vi "test.vi"() -> ()   [LabVIEW 2012]
panel:
  out "x/y":sgl
  in  "数值 2":sgl
  in  "数值":sgl
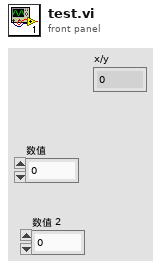
[diagram p1: front panel]
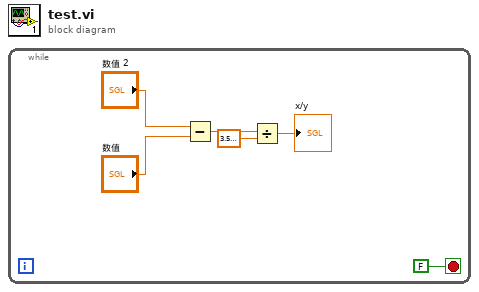
[diagram p0: block diagram]
diagram:
  n1 = while {
    stop <- FALSE stop-if-true
    n2 = Subtract(x="数值 2", y="数值") -> (x-y=w3:sgl)
    n3 = Divide(x=w3, y=sgl 3.6) -> (x/y=→"x/y":sgl)
  }
